vi "Example (R Series).vi"() -> ()   [LabVIEW 2010]
uses:
  <vilib>/eio/EIONode/EIONode.xnode
panel:
  in  "Wait (Milliseconds)":u32
  out "Device Temperature":i16
  in  "Stop":bool
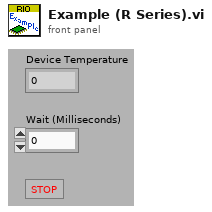
[diagram p1: front panel]
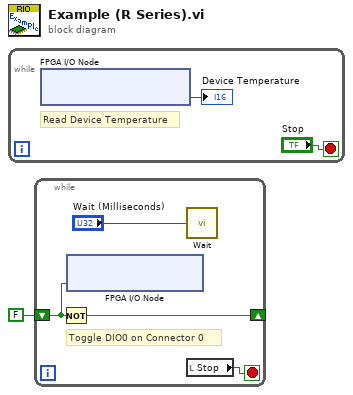
[diagram p0: block diagram]
diagram:
  n1 = while {
    stop <- "Stop" stop-if-true
    # "Read Device Temperature"
    n2 = xnode "FPGA I/O Node"() -> ("Device Temperature"=→"Device Temperature":i16)  [unwired: 1 in, 1 out]
  }
  n3 = while {
    shift-right: [w5] -> _
    shift-left: FALSE ("stop") -> [w6]
    stop <- w7 stop-if-true
    # "Toggle DIO0 on Connector 0"
    n4 = Not(x=w6) -> (.not. x?=w5:bool)
    n5 = xnode "FPGA I/O Node"("Connector0/DIO0"=w6) -> ()  [unwired: 1 in, 1 out]
    n6 = call "Wait"("Count(mSec)"="Wait (Milliseconds)") -> ()  [unwired: 1 out]
    n7 = local read "Stop"() -> (w7:bool)
  }
